vi "Test RE.vi"() -> ()   [LabVIEW 2013]
uses:
  <vilib>/regexp/Match Regular Expression.xnode
panel:
  out "submatch 5":string
  out "submatch 4":string
  out "submatch 3":string
  out "submatch 2":string
  out "after substring":string
  out "match substring":string
  out "before substring":string
  in  "regular expression":string="version ([0-9]+\\.[0-9]+\\.[0-9]+)"
  out "submatch 1":string
  in  "input string":string
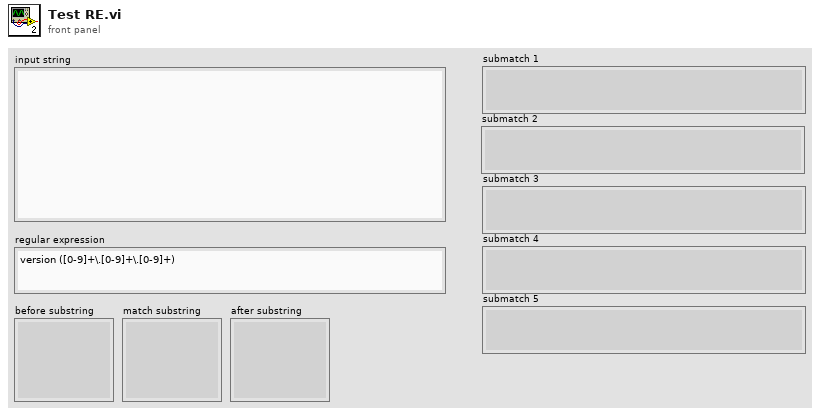
[diagram p1: front panel]
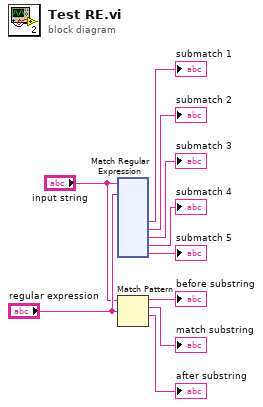
[diagram p0: block diagram]
diagram:
  n1 = xnode "Match Regular Expression"("input string"="input string", "regular expression"="regular expression") -> ("submatch 1"=→"submatch 1":string, "submatch 2"=→"submatch 2":string, "submatch 3"=→"submatch 3":string, "submatch 4"=→"submatch 4":string, "submatch 5"=→"submatch 5":string)  [unwired: 4 in, 5 out]
  n2 = Match Pattern(string="input string", regular expression="regular expression") -> (before substring=→"before substring":string, match substring=→"match substring":string, after substring=→"after substring":string)  [unwired: 1 in, 1 out]
